vi "form_slope.vi"(11 "JSON":string="{\"cmd\":\"set_feedback\",\"args\":{\"fb channel\":0, \"fb config\":{\"Setpoint\":1, \"Output limit (low)\":-5, \"Output limit (high)\":10, \"P gain\":1e-3, \"I gain\":1e-3, \"Reset\":true, \"Hold\":false, \"Negative\":true, \"Input channel\":0, \"Output channel\":2, \"wait for fb\":false, \"Error limit (high)\":0.1, \"Error limit (low)\":-0.1}}}") -> ()   [LabVIEW 2020]
doc: "Form template VI.\n\nWhen you want to create a new form, please copy and modify this VI.\nThe form vi should be placed in the host/form directory."
uses:
  core/host_global_vars.vi
  <vilib>/rvi/interface/RandomDataEmulation/niFpgaReadControlTemplate.vi
  <vilib>/rvi/interface/RandomDataEmulation/niFpgaWriteControlTemplate.vi
  <vilib>/rvi/interface/nirviReadWriteControl/nirviReadWriteControl.xnode
  fpga/fpga_main.vi
panel:
  in  "slope":cluster{"x":sgl, "y":sgl} {"x" scale=-1.0..1.0; "y" scale=-1.0..1.0}
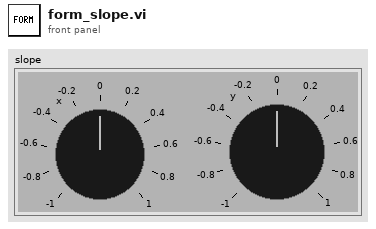
[diagram p1: front panel]
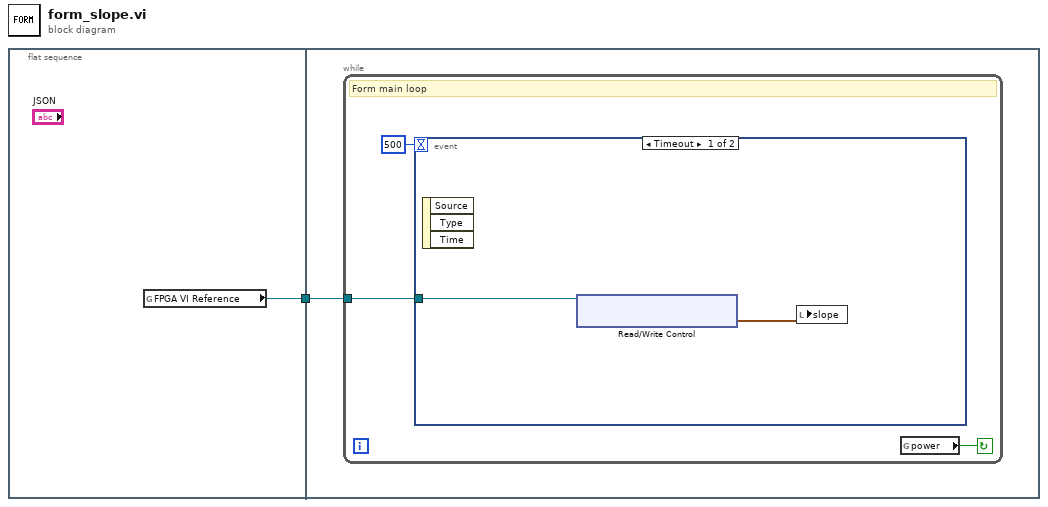
[diagram p0: block diagram]
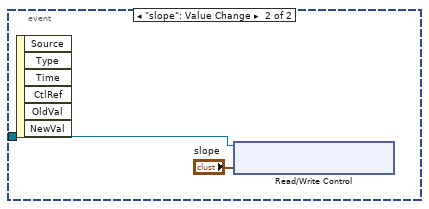
[diagram p2: hidden frame]
diagram:
  n1 = flat-sequence {
    tunnel: [w2] -> w1
    tunnel: w1 -> [w3]
    frame #0 {
      n2 = global read "host_global_vars.vi" "FPGA VI Reference"() -> (w2:refnum<k20>)
    }
    frame #1 {
      n3 = while {
        tunnel: w3 -> [w5]
        stop <- w6 continue-if-true
        # "Form main loop"
        n4 = event shown="[0] Timeout" {
          selector: _ -> [_ _]
          dyn-events: _ -> [_ _]
          timeout: 500 -> [_ _]
          tunnel: w5 -> [w8 w10]
          event Timeout {
            n5 = event-data() -> ()  [unwired: 1 in, 3 out]
            n6 = xnode "Read/Write Control"("FPGA VI Reference In"=w8) -> ("slope"=w7:cluster{"x":sgl, "y":sgl})  [unwired: 1 in, 2 out]
            n7 = local write "slope"(w7) -> ()
          }
          event "slope": Value Change {
            n8 = event-data() -> ()  [unwired: 1 in, 6 out]
            n9 = xnode "Read/Write Control"("FPGA VI Reference In"=w10, "slope"="slope") -> ()  [unwired: 1 in, 2 out]
          }
        }
        n10 = global read "host_global_vars.vi" "power"() -> (w6:bool)
      }
    }
  }
